vi "0926New Project.vi"() -> ()   [LabVIEW 2011] (continued)
      n72 = property on="S-para Pair Name" class="LstBox (严格)"("Value"=w56) -> ()  [unwired: 2 in, 2 out]
      n73 = property on="NEXT Pair Name" class="LstBox (严格)"("Value"=w56) -> ()  [unwired: 2 in, 2 out]
      n74 = property on="FEXT Pair Name" class="LstBox (严格)"("Value"=w56) -> ()  [unwired: 2 in, 2 out]
      n75 = property on="Single Test Items" class="LstBox (严格)"("Value"=w56) -> ()  [unwired: 2 in, 2 out]
      n76 = property on="FEXT Pair Name" class="LstBox (严格)"("Value"=w56) -> ()  [unwired: 2 in, 2 out]
      n77 = property on="Cable AWG:" class="Ring (严格)"("Value"=w56) -> ()  [unwired: 2 in, 2 out]
      n78 = property on="Customer" class="Ring (严格)"("Value"=w56) -> ()  [unwired: 2 in, 2 out]
      n79 = property on="TDR Test Items" class="LstBox (严格)"("Value"=w56) -> ()  [unwired: 2 in, 2 out]
      n80 = call <vilib>:"Application Directory.vi"() -> ("Application Directory"=w32:path)
      n81 = property on="Default" class="RadioBtnsControl (严格)"("Value"=w56) -> ()  [unwired: 2 in, 2 out]
      n82 = Build Path(base path=w32, name or relative path="template" ("名称或相对路径")) -> (appended path=w33:path)
      n83 = call "Get_initialize_Config.vi"() -> ("Local Database"=w24:bool)  [unwired: 11 in]
      n84 = local write "Report Templete Path:"(w33) -> ()
      n85 = local write "Local"(w24) -> ()
      n86 = property on="Excute" class="Bool"("DisabledEnum"=w29) -> ()  [unwired: 2 in, 2 out]
      n87 = property on="Query" class="Bool (严格)"("DisabledEnum"=w29) -> ()  [unwired: 2 in, 2 out]
      n88 = property on="Save" class="Bool (严格)"("DisabledEnum"=T4."Disabled and Grayed Out" ("禁用")) -> ()  [unwired: 2 in, 2 out]
      n89 = local write "Query"(FALSE ("Query")) -> ()
      n90 = local write "Update"(FALSE ("Query")) -> ()
      n91 = local write "Delete"(FALSE ("Query")) -> ()
      n92 = local write "Save"(FALSE ("Query")) -> ()
      n93 = property on="SNType" class="Str"("Visible"=w24) -> ()  [unwired: 2 in, 2 out]
      n94 = property on="CmdType" class="Ring (严格)"("Visible"=w24) -> ()  [unwired: 2 in, 2 out]
      n95 = property on="Update" class="Bool (严格)"("DisabledEnum"=T4."Disabled and Grayed Out" ("禁用")) -> ()  [unwired: 2 in, 2 out]
      n96 = property on="Delete" class="Bool (严格)"("DisabledEnum"=T4."Disabled and Grayed Out" ("禁用")) -> ()  [unwired: 2 in, 2 out]
      n97 = property on="Luxshare_P/N:" class="Str"("DisabledEnum"=T4."Disabled and Grayed Out" ("禁用")) -> ()  [unwired: 2 in, 2 out]
      "midVar_bool_timStop" <- FALSE ("midVar_bool_timStop")
    }
    frame #2 {
      n98 = while {
        stop <- w104 stop-if-true
        n99 = local read "midVar_timeStart"() -> (w103:timestamp)
        n100 = local read "midVar_bool_timStop"() -> (w104:bool)
        n101 = Get Date/Time In Seconds() -> (seconds since 1Jan1904=w105:timestamp)
        n102 = Subtract(x=w105, y=w103) -> (x-y=→"访问DB(s)":dbl)
      }
      n103 = call <vilib>:"System Exec.vi"("run minimized? (F)"=TRUE, "wait until completion? (T)"=TRUE, "command line"="ping DG-MESDB.luxshare.com.cn") -> ("standard output"=w96:string)  [unwired: 5 in, 3 out]
      n104 = Search and Replace String(replace all?=TRUE ("替换全部？(F)"), case sensitive?=TRUE ("忽略大小写？(F)"), input string=w96, search string="TTL" ("搜索字符串")) -> (number of replacements=w98:i32)  [unwired: 4 in, 3 out]
      n105 = Greater Than 0?(x=w98) -> (x > 0?=w93:bool)
      n106 = case shown="真" w93 {
        frame False {
          w109 = T4."Enabled" ("禁用")
          # "连不上数据库，local禁用，默认勾选"
          n107 = property on="Query" class="Bool (严格)"("DisabledEnum"=w109) -> ()  [unwired: 2 in, 2 out]
          n108 = property on="Save" class="Bool (严格)"("DisabledEnum"=w109) -> ()  [unwired: 2 in, 2 out]
          n109 = local write "midVar_bool_timStop"(TRUE ("midVar_bool_timStop")) -> ()
          n110 = One Button Dialog(message="fail to connect DB!\nyou can use local DB only!") -> ()  [unwired: 1 in, 1 out]
          n111 = property on="Excute" class="Bool"("DisabledEnum"=w109) -> ()  [unwired: 2 in, 2 out]
          n112 = property on="Local" class="Bool (严格)"("DisabledEnum"=T4."Disabled and Grayed Out" ("禁用")) -> ()  [unwired: 2 in, 2 out]
          n113 = local write "Local"(TRUE ("Local")) -> ()
          n114 = property on="FixtureNo" class="CmbBox"("Strings And Values[]"=T5 [{"String"="No Data", "Value"="No Data"}] ("字符串与值[]")) -> ()  [unwired: 2 in, 2 out]
          n115 = property on="FixtureNo" class="CmbBox"("DisabledEnum"=T4."Disabled and Grayed Out" ("禁用")) -> ()  [unwired: 2 in, 2 out]
        }
        frame True {
          n116 = stacked-sequence {
            frame #0 {
              w114 = T4."Enabled" ("禁用")
              w113 = T4."Enabled" ("禁用")
              n117 = property on="Local" class="Bool (严格)"("DisabledEnum"=w113) -> ()  [unwired: 2 in, 2 out]
              n118 = property on="Query" class="Bool (严格)"("DisabledEnum"=w113) -> ()  [unwired: 2 in, 2 out]
              n119 = property on="Save" class="Bool (严格)"("DisabledEnum"=w114) -> ()  [unwired: 2 in, 2 out]
              n120 = property on="Excute" class="Bool"("DisabledEnum"=w114) -> ()  [unwired: 2 in, 2 out]
            }
            frame #1 {
              n121 = call "sql-readinfo_vfixture.vi"("操作模式"=T6."查询数据", "查询项目"="FixtureNo", "限定条件"="") -> ("ConvertToArray"=w119:string[][], "ResultString"=w118:string)  [unwired: 14 in, 9 out]
              n122 = call <vilib>:"Trim Whitespace.vi"("string"=w118) -> ("trimmed string"=w117:string)  [unwired: 1 in]
              n123 = Empty String/Path?(string/path=w117) -> (empty?=w116:bool)
              n124 = case shown="假" w116 {
                tunnel: w119 -> [w126 _]
                frame False {
                  n125 = Index Array(array=w126, index (col)=0 ("索引 (行)")) -> (element=w125:string[])  [unwired: 1 in]
                  n126 = for {
                    tunnel: w125 -> [w128] mode=indexing
                    tunnel: [w127] -> w124 mode=indexing
                    n127 = Bundle("字符串"=w128, "字符串"=w128) -> (w127:cluster{"字符串":string, "字符串":string})  [unwired: 1 in]
                  }
                  n128 = property on="FixtureNo" class="CmbBox"("Strings And Values[]"=w124) -> ()  [unwired: 2 in, 2 out]
                  n129 = property on="FixtureNo" class="CmbBox"("DisabledEnum"=T4."Enabled" ("禁用")) -> ()  [unwired: 2 in, 2 out]
                }
                frame True {
                  n130 = property on="FixtureNo" class="CmbBox"("Strings And Values[]"=T5 [{"String"="No Data", "Value"="No Data"}] ("字符串与值[]")) -> ()  [unwired: 2 in, 2 out]
                  n131 = property on="FixtureNo" class="CmbBox"("DisabledEnum"=T4."Disabled and Grayed Out" ("禁用")) -> ()  [unwired: 2 in, 2 out]
                }
              }
            }
            frame #2 {
              n132 = local write "midVar_bool_timStop"(TRUE ("midVar_bool_timStop")) -> ()
            }
          }
        }
      }
    }
    frame #3 {
      n133 = control-ref of="Label Num"() -> (w132:refnum<vi>)
      n134 = control-ref of="FixtureNo"() -> (w155:refnum<vi>)
      n135 = control-ref of="Label Num"() -> (w154:refnum<vi>)
      n136 = control-ref of="Label Content"() -> (w153:refnum<vi>)
      n137 = control-ref of="SNType"() -> (w152:refnum<vi>)
      n138 = control-ref of="Customer_P/N:"() -> (w162:refnum<vi>)
      n139 = control-ref of="Length(mm):"() -> (w161:refnum<vi>)
      n140 = control-ref of="Sample Description:"() -> (w160:refnum<vi>)
      n141 = control-ref of="Remark:"() -> (w159:refnum<vi>)
      n142 = control-ref of="Switch Matrix"() -> (w158:refnum<vi>)
      n143 = control-ref of="VNA Cal File Path:"() -> (w156:refnum<vi>)
      n144 = control-ref of="EEPROM Write/Read ?"() -> (w151:refnum<vi>)
      n145 = control-ref of="Label Print?"() -> (w150:refnum<vi>)
      n146 = Build Array(w151, w150) -> (→"bool":refnum<vi>[])
      n147 = Build Array(w156, w162, w161, w160, w159, w158, w155, w154, w153, w132, w152) -> (→"string":refnum<vi>[])
      n148 = control-ref of="Spec Associate"() -> (w148:refnum<vi>)
      n149 = control-ref of="Postion for Raw data"() -> (w147:refnum<vi>)
      n150 = control-ref of="Impedance Spec:"() -> (w133:refnum<vi>)
      n151 = control-ref of="Start TimeNs"() -> (w146:refnum<vi>)
      n152 = control-ref of="StopTimeNs"() -> (w145:refnum<vi>)
      n153 = control-ref of="Filter Risetime(ps)"() -> (w144:refnum<vi>)
      n154 = control-ref of="Compensation(ohm)"() -> (w143:refnum<vi>)
      n155 = Build Array(w133, w148, w147) -> (→"chart":refnum<vi>[])
      n156 = Build Array(w146, w145, w144, w143) -> (→"number":refnum<vi>[])
      n157 = control-ref of="Diff Test Items"() -> (w142:refnum<vi>)
      n158 = control-ref of="Single Test Items"() -> (w141:refnum<vi>)
      n159 = control-ref of="TDR Test Items"() -> (w140:refnum<vi>)
      n160 = control-ref of="S-para Pair Name"() -> (w139:refnum<vi>)
      n161 = control-ref of="NEXT Pair Name"() -> (w138:refnum<vi>)
      n162 = control-ref of="FEXT Pair Name"() -> (w137:refnum<vi>)
      n163 = Build Array(w142, w141, w140, w139, w138, w137) -> (→"list":refnum<vi>[])
      n164 = property on="访问DB(s)" class="DigNum (严格)"("Visible"=FALSE ("可见")) -> ()  [unwired: 2 in, 2 out]
    }
    frame #4 {
      n165 = while {
        stop <- w165 stop-if-true
        n166 = event shown="[17] \"Excute\": 值改变" {
          selector: _ -> [_ _ _ _ _ _ _ _ _ _ _ _ _ _ _ _ _ _ _ _ _ _ _]
          dyn-events: _ -> [_ _ _ _ _ _ _ _ _ _ _ _ _ _ _ _ _ _ _ _ _ _ _]
          timeout: 500 -> [_ _ _ _ _ _ _ _ _ _ _ _ _ _ _ _ _ _ _ _ _ _ _]
          tunnel: [_ _ _ _ _ _ _ _ _ _ _ _ _ _ _ _ _ _ _ TRUE _ _ _] -> w165
          event Timeout {
            n167 = event-data() -> ()  [unwired: 1 in, 2 out]
          }
          event "Length(mm):", "VNA Cal File Path:", "Switch Matrix", "Luxshare_P/N:": Value Change {
            n168 = event-data() -> ()  [unwired: 1 in, 5 out]
          }
          event "Local": Value Change {
            n169 = event-data() -> ()  [unwired: 1 in, 5 out]
            n170 = local read "Local"() -> (w166:bool)
            n171 = Not(x=w166) -> (.not. x?=w167:bool)
            n172 = property on="SNType" class="Str"("Visible"=w166) -> ()  [unwired: 2 in, 2 out]
            n173 = property on="CmdType" class="Ring (严格)"("Visible"=w166) -> ()  [unwired: 2 in, 2 out]
            n174 = property on="System_Mode" class="Ring (严格)"("Visible"=w167) -> ()  [unwired: 2 in, 2 out]
          }
          event "Quick": Value Change {
            n175 = event-data() -> ("NewVal"=w170:bool)  [unwired: 1 in, 4 out]
            n176 = Equal?(x=w170, y=TRUE) -> (x = y?=w168:bool)
            n177 = case shown="真" w168 {
              frame False {
                n178 = property on="Postion for Raw data" class="Tbl (严格)"("Value"=string[][] [] ("Postion for Raw data")) -> ()  [unwired: 2 in, 2 out]
              }
              frame True {
                w173 = T3 {"Row"=0, "Column"=0} ("编辑位置")
                w174 = u32 4 ("列数")
                n179 = property on="Single Test Items" class="LstBox (严格)"() -> ("Item Names"=w191:string[], "Item Symbols"=w190:i32[])  [unwired: 2 in, 2 out]
                n180 = property on="TDR Test Items" class="LstBox (严格)"() -> ("Item Names"=w189:string[], "Item Symbols"=w188:i32[])  [unwired: 2 in, 2 out]
                n181 = property on="Diff Test Items" class="LstBox (严格)"() -> ("Item Names"=w193:string[], "Item Symbols"=w192:i32[])  [unwired: 2 in, 2 out]
                n182 = call "_wmg_SelectItems2.vi"("Item Syms"=w188, "Item name"=w189) -> ("Selected tem"=w187:string[])  [unwired: 7 in, 2 out]
                n183 = call "_wmg_SelectItems2.vi"("Item Syms"=w192, "Item name"=w193) -> ("Selected tem"=w186:string[])  [unwired: 7 in, 2 out]
                n184 = call "_wmg_SelectItems2.vi"("Item Syms"=w190, "Item name"=w191) -> ("Selected tem"=w185:string[])  [unwired: 7 in, 2 out]
                n185 = Insert Into Array(array=w187, new element #1=w186, new element #2=w185) -> (w182:string[])  [unwired: 1 in]
                n186 = Array Size(array=w182) -> (size(s)=w179:i32)
                n187 = for {
                  N: w179 -> [_]
                  tunnel: [w194] -> w183 mode=indexing
                  i -> [w195]
                  n188 = Increment(x=w195) -> (x+1=w194:i32)
                }
                n189 = Initialize Array("2", w179) -> (w177:string[])
                n190 = Initialize Array("0", w179) -> (w176:string[])
                n191 = Number To Decimal String(number=w183) -> (decimal integer string=w181:string[])  [unwired: 1 in]
                n192 = Build Array(w182, w181, w177, w176) -> (w175:string[][])
                n193 = Transpose 2D Array(2D array=w175) -> (transposed array=w184:string[][])
                n194 = property on="Postion for Raw data" class="Tbl (严格)"("Value"=w184, "EditPos"=T3 {"Row"=0, "Column"=0} ("编辑位置")) -> ()  [unwired: 2 in, 2 out]
                n195 = property on="Postion for Raw data" class="Tbl (严格)"("Number of Columns"=w174, "EditPos"=w173) -> ()  [unwired: 2 in, 2 out]
                n196 = property on="Postion for \"PN&Tester&Date\" etc Fields" class="Tbl (严格)"("Number of Columns"=w174, "EditPos"=w173) -> ()  [unwired: 2 in, 2 out]
              }
            }
          }
          event "Diff Test Items": Double Click {
            n197 = event-data() -> ("Row"=w196:i32)  [unwired: 1 in, 7 out]
            n198 = stacked-sequence {
              tunnel: w196 -> [w203 _ _]
              frame #0 {
                w200 = 38 ("y")
                n199 = property on="Diff Test Items" class="LstBox (严格)"() -> ("Item Symbols"=w204:i32[])  [unwired: 2 in, 2 out]
                n200 = Index Array(array=w204, index=w203) -> (element=w202:i32)
                n201 = Equal?(x=w202, y=w200) -> (x = y?=w201:bool)
                n202 = Select(t=37, s=w201, f=w200) -> (s? t:f=w198:i32)
                n203 = Replace Array Subset(array=w204, new element=w198, index=w203) -> (w197:i32[])
                n204 = property on="Diff Test Items" class="LstBox (严格)"("Item Symbols"=w197) -> ()  [unwired: 2 in, 2 out]
              }
              frame #1 {
                n205 = property on="Postion for Raw data" class="Tbl (严格)"("Value"=string[][] [] ("Postion for Raw data"), "EditPos"=T3 {"Row"=0, "Column"=0} ("编辑位置")) -> ()  [unwired: 2 in, 2 out]
              }
              frame #2 {
                w208 = T3 {"Row"=0, "Column"=0} ("编辑位置")
                w209 = u32 4 ("列数")
                n206 = property on="Single Test Items" class="LstBox (严格)"() -> ("Item Names"=w226:string[], "Item Symbols"=w225:i32[])  [unwired: 2 in, 2 out]
                n207 = property on="TDR Test Items" class="LstBox (严格)"() -> ("Item Names"=w224:string[], "Item Symbols"=w223:i32[])  [unwired: 2 in, 2 out]
                n208 = property on="Diff Test Items" class="LstBox (严格)"() -> ("Item Names"=w228:string[], "Item Symbols"=w227:i32[])  [unwired: 2 in, 2 out]
                n209 = property on="Postion for Raw data" class="Tbl (严格)"("Number of Columns"=w209, "EditPos"=w208) -> ()  [unwired: 2 in, 2 out]
                n210 = property on="Postion for \"PN&Tester&Date\" etc Fields" class="Tbl (严格)"("Number of Columns"=w209, "EditPos"=w208) -> ()  [unwired: 2 in, 2 out]
                n211 = call "_wmg_SelectItems2.vi"("Item Syms"=w223, "Item name"=w224) -> ("Selected tem"=w222:string[])  [unwired: 7 in, 2 out]
                n212 = call "_wmg_SelectItems2.vi"("Item Syms"=w227, "Item name"=w228) -> ("Selected tem"=w221:string[])  [unwired: 7 in, 2 out]
                n213 = call "_wmg_SelectItems2.vi"("Item Syms"=w225, "Item name"=w226) -> ("Selected tem"=w220:string[])  [unwired: 7 in, 2 out]
                n214 = Insert Into Array(array=w222, new element #1=w221, new element #2=w220) -> (w217:string[])  [unwired: 1 in]
                n215 = Array Size(array=w217) -> (size(s)=w214:i32)
                n216 = for {
                  N: w214 -> [_]
                  tunnel: [w229] -> w218 mode=indexing
                  i -> [w230]
                  n217 = Increment(x=w230) -> (x+1=w229:i32)
                }
                n218 = Initialize Array("2", w214) -> (w212:string[])
                n219 = Initialize Array("0", w214) -> (w211:string[])
                n220 = Number To Decimal String(number=w218) -> (decimal integer string=w216:string[])  [unwired: 1 in]
                n221 = Build Array(w217, w216, w212, w211) -> (w210:string[][])
                n222 = Transpose 2D Array(2D array=w210) -> (transposed array=w219:string[][])
                n223 = property on="Postion for Raw data" class="Tbl (严格)"("Value"=w219, "EditPos"=T3 {"Row"=0, "Column"=0} ("编辑位置")) -> ()  [unwired: 2 in, 2 out]
              }
            }
          }
          event "TDR Test Items": Double Click {
            n224 = event-data() -> ("Row"=w231:i32)  [unwired: 1 in, 7 out]
            n225 = stacked-sequence {
              tunnel: w231 -> [w239 _ _]
              frame #0 {
                w236 = 38 ("y")
                n226 = property on="TDR Test Items" class="LstBox (严格)"() -> ("Item Symbols"=w233:i32[])  [unwired: 2 in, 2 out]
                n227 = Index Array(array=w233, index=w239) -> (element=w238:i32)
                n228 = Equal?(x=w238, y=w236) -> (x = y?=w237:bool)
                n229 = Select(t=37, s=w237, f=w236) -> (s? t:f=w234:i32)
                n230 = Replace Array Subset(array=w233, new element=w234, index=w239) -> (w232:i32[])
                n231 = property on="TDR Test Items" class="LstBox (严格)"("Item Symbols"=w232) -> ()  [unwired: 2 in, 2 out]
              }
              frame #1 {
                n232 = property on="Postion for Raw data" class="Tbl (严格)"("Value"=string[][] [] ("Postion for Raw data"), "EditPos"=T3 {"Row"=0, "Column"=0} ("编辑位置")) -> ()  [unwired: 2 in, 2 out]
              }
              frame #2 {
                w243 = T3 {"Row"=0, "Column"=0} ("编辑位置")
                w244 = u32 4 ("列数")
                n233 = property on="Single Test Items" class="LstBox (严格)"() -> ("Item Names"=w261:string[], "Item Symbols"=w260:i32[])  [unwired: 2 in, 2 out]
                n234 = property on="TDR Test Items" class="LstBox (严格)"() -> ("Item Names"=w259:string[], "Item Symbols"=w258:i32[])  [unwired: 2 in, 2 out]
                n235 = property on="Diff Test Items" class="LstBox (严格)"() -> ("Item Names"=w263:string[], "Item Symbols"=w262:i32[])  [unwired: 2 in, 2 out]
                n236 = property on="Postion for Raw data" class="Tbl (严格)"("Number of Columns"=w244, "EditPos"=w243) -> ()  [unwired: 2 in, 2 out]
                n237 = property on="Postion for \"PN&Tester&Date\" etc Fields" class="Tbl (严格)"("Number of Columns"=w244, "EditPos"=w243) -> ()  [unwired: 2 in, 2 out]
                n238 = call "_wmg_SelectItems2.vi"("Item Syms"=w258, "Item name"=w259) -> ("Selected tem"=w257:string[])  [unwired: 7 in, 2 out]
                n239 = call "_wmg_SelectItems2.vi"("Item Syms"=w262, "Item name"=w263) -> ("Selected tem"=w256:string[])  [unwired: 7 in, 2 out]
                n240 = call "_wmg_SelectItems2.vi"("Item Syms"=w260, "Item name"=w261) -> ("Selected tem"=w255:string[])  [unwired: 7 in, 2 out]
                n241 = Insert Into Array(array=w257, new element #1=w256, new element #2=w255) -> (w252:string[])  [unwired: 1 in]
                n242 = Array Size(array=w252) -> (size(s)=w249:i32)
                n243 = for {
                  N: w249 -> [_]
                  tunnel: [w264] -> w253 mode=indexing
                  i -> [w265]
                  n244 = Increment(x=w265) -> (x+1=w264:i32)
                }
                n245 = Initialize Array("2", w249) -> (w247:string[])
                n246 = Initialize Array("0", w249) -> (w246:string[])
                n247 = Number To Decimal String(number=w253) -> (decimal integer string=w251:string[])  [unwired: 1 in]
                n248 = Build Array(w252, w251, w247, w246) -> (w245:string[][])
                n249 = Transpose 2D Array(2D array=w245) -> (transposed array=w254:string[][])
                n250 = property on="Postion for Raw data" class="Tbl (严格)"("Value"=w254, "EditPos"=T3 {"Row"=0, "Column"=0} ("编辑位置")) -> ()  [unwired: 2 in, 2 out]
              }
            }
          }
          event "S-para Pair Name": Double Click {
            w270 = 38 ("y")
            n251 = event-data() -> ("Row"=w266:i32)  [unwired: 1 in, 7 out]
            n252 = property on="S-para Pair Name" class="LstBox (严格)"() -> ("Item Symbols"=w273:i32[])  [unwired: 2 in, 2 out]
            n253 = Index Array(array=w273, index=w266) -> (element=w272:i32)
            n254 = Equal?(x=w272, y=w270) -> (x = y?=w271:bool)
            n255 = Select(t=37, s=w271, f=w270) -> (s? t:f=w268:i32)
            n256 = Replace Array Subset(array=w273, new element=w268, index=w266) -> (w267:i32[])
            n257 = property on="S-para Pair Name" class="LstBox (严格)"("Item Symbols"=w267) -> ()  [unwired: 2 in, 2 out]
          }
          event "NEXT Pair Name": Double Click {
            w278 = 38 ("y")
            n258 = event-data() -> ("Row"=w274:i32)  [unwired: 1 in, 7 out]
            n259 = property on="NEXT Pair Name" class="LstBox (严格)"() -> ("Item Symbols"=w281:i32[])  [unwired: 2 in, 2 out]
            n260 = Index Array(array=w281, index=w274) -> (element=w280:i32)
            n261 = Equal?(x=w280, y=w278) -> (x = y?=w279:bool)
            n262 = Select(t=37, s=w279, f=w278) -> (s? t:f=w276:i32)
            n263 = Replace Array Subset(array=w281, new element=w276, index=w274) -> (w275:i32[])
            n264 = property on="NEXT Pair Name" class="LstBox (严格)"("Item Symbols"=w275) -> ()  [unwired: 2 in, 2 out]
          }
          event "FEXT Pair Name": Double Click {
            w282 = 38 ("y")
            n265 = event-data() -> ("Row"=w283:i32)  [unwired: 1 in, 7 out]
            n266 = property on="FEXT Pair Name" class="LstBox (严格)"() -> ("Item Symbols"=w289:i32[])  [unwired: 2 in, 2 out]
            n267 = Index Array(array=w289, index=w283) -> (element=w288:i32)
            n268 = Equal?(x=w288, y=w282) -> (x = y?=w287:bool)
            n269 = Select(t=37, s=w287, f=w282) -> (s? t:f=w285:i32)
            n270 = Replace Array Subset(array=w289, new element=w285, index=w283) -> (w284:i32[])
            n271 = property on="FEXT Pair Name" class="LstBox (严格)"("Item Symbols"=w284) -> ()  [unwired: 2 in, 2 out]
          }
          event "Single Test Items": Double Click {
            n272 = event-data() -> ("Row"=w290:i32)  [unwired: 1 in, 7 out]
            n273 = stacked-sequence {
              tunnel: w290 -> [w292 _ _]
              frame #0 {
                w291 = 38 ("y")
                n274 = property on="Single Test Items" class="LstBox (严格)"() -> ("Item Symbols"=w298:i32[])  [unwired: 2 in, 2 out]
                n275 = Index Array(array=w298, index=w292) -> (element=w297:i32)
                n276 = Equal?(x=w297, y=w291) -> (x = y?=w296:bool)
                n277 = Select(t=37, s=w296, f=w291) -> (s? t:f=w294:i32)
                n278 = Replace Array Subset(array=w298, new element=w294, index=w292) -> (w293:i32[])
                n279 = property on="Single Test Items" class="LstBox (严格)"("Item Symbols"=w293) -> ()  [unwired: 2 in, 2 out]
              }
              frame #1 {
                n280 = property on="Postion for Raw data" class="Tbl (严格)"("Value"=string[][] [] ("Postion for Raw data"), "EditPos"=T3 {"Row"=0, "Column"=0} ("编辑位置")) -> ()  [unwired: 2 in, 2 out]
              }
              frame #2 {
                w302 = T3 {"Row"=0, "Column"=0} ("编辑位置")
                w303 = u32 4 ("列数")
                n281 = property on="Single Test Items" class="LstBox (严格)"() -> ("Item Names"=w320:string[], "Item Symbols"=w319:i32[])  [unwired: 2 in, 2 out]
                n282 = property on="TDR Test Items" class="LstBox (严格)"() -> ("Item Names"=w318:string[], "Item Symbols"=w317:i32[])  [unwired: 2 in, 2 out]
                n283 = property on="Diff Test Items" class="LstBox (严格)"() -> ("Item Names"=w322:string[], "Item Symbols"=w321:i32[])  [unwired: 2 in, 2 out]
                n284 = property on="Postion for Raw data" class="Tbl (严格)"("Number of Columns"=w303, "EditPos"=w302) -> ()  [unwired: 2 in, 2 out]
                n285 = property on="Postion for \"PN&Tester&Date\" etc Fields" class="Tbl (严格)"("Number of Columns"=w303, "EditPos"=w302) -> ()  [unwired: 2 in, 2 out]
                n286 = call "_wmg_SelectItems2.vi"("Item Syms"=w317, "Item name"=w318) -> ("Selected tem"=w316:string[])  [unwired: 7 in, 2 out]
                n287 = call "_wmg_SelectItems2.vi"("Item Syms"=w321, "Item name"=w322) -> ("Selected tem"=w315:string[])  [unwired: 7 in, 2 out]
                n288 = call "_wmg_SelectItems2.vi"("Item Syms"=w319, "Item name"=w320) -> ("Selected tem"=w314:string[])  [unwired: 7 in, 2 out]
                n289 = Insert Into Array(array=w316, new element #1=w315, new element #2=w314) -> (w311:string[])  [unwired: 1 in]
                n290 = Array Size(array=w311) -> (size(s)=w308:i32)
                n291 = for {
                  N: w308 -> [_]
                  tunnel: [w323] -> w312 mode=indexing
                  i -> [w324]
                  n292 = Increment(x=w324) -> (x+1=w323:i32)
                }
                n293 = Initialize Array("2", w308) -> (w306:string[])
                n294 = Initialize Array("0", w308) -> (w305:string[])
                n295 = Number To Decimal String(number=w312) -> (decimal integer string=w310:string[])  [unwired: 1 in]
                n296 = Build Array(w311, w310, w306, w305) -> (w304:string[][])
                n297 = Transpose 2D Array(2D array=w304) -> (transposed array=w313:string[][])
                n298 = property on="Postion for Raw data" class="Tbl (严格)"("Value"=w313, "EditPos"=T3 {"Row"=0, "Column"=0} ("编辑位置")) -> ()  [unwired: 2 in, 2 out]
              }
            }
          }
          event "Import Spec": Value Change {
            n299 = event-data() -> ()  [unwired: 1 in, 5 out]
            n300 = case shown="真" "Import Spec" {
              frame False {
              }
              frame True {
                n301 = call <vilib>:"Application Directory.vi"() -> ("Application Directory"=w328:path)
                n302 = Build Path(base path=w328, name or relative path="Spec" ("名称或相对路径")) -> (appended path=w326:path)
                n303 = call "文件对话框"("start path"=w326) -> ("selected path"=w330:path, "error out"=w329:errorcluster)  [unwired: 11 in, 2 out]
                n304 = case shown="无错误" w329 {
                  tunnel: w330 -> [w331 _]
                  frame No Error {
                    n305 = stacked-sequence {
                      tunnel: w331 -> [_ w359]
                      frame #0 {
                        n306 = property on="Diff Test Items" class="LstBox (严格)"() -> ("Item Symbols"=w338:i32[], "Item Names"=w336:string[])  [unwired: 2 in, 2 out]
                        n307 = for {
                          tunnel: w338 -> [w349] mode=indexing
                          shift-right: [w344] -> w334
                          shift-left: string[] [] -> [w345]
                          tunnel: w336 -> [w346] mode=indexing
                          shift-right: [w343] -> w333
                          shift-left: string[] [] -> [w342]
                          n308 = Array Size(array=w342) -> (size(s)=w341:i32)
                          n309 = Equal?(x=w349, y=38) -> (x = y?=w347:bool)
                          n310 = Increment(x=w341) -> (x+1=w340:i32)
                          n311 = Number To Decimal String(number=w340) -> (decimal integer string=w339:string)  [unwired: 1 in]
                          n312 = case shown="真" w347 {
                            tunnel: w346 -> [_ w357]
                            tunnel: w345 -> [w351 w356]
                            tunnel: [w351 w355] -> w344
                            tunnel: w342 -> [w350 w354]
                            tunnel: [w350 w353] -> w343
                            tunnel: w339 -> [_ w352]
                            frame False {
                            }
                            frame True {
                              n313 = Insert Into Array(array=w354, new element=w352) -> (w353:string[])  [unwired: 1 in]
                              n314 = Insert Into Array(array=w356, new element=w357) -> (w355:string[])  [unwired: 1 in]
                            }
                          }
                        }
                        n315 = Build Array(w334, w333) -> (w332:string[][])
                        n316 = local write "Spec Associate"(w332) -> ()
                      }
                      frame #1 {
                        n317 = Path To String(path=w359) -> (string=w358:string)
                        n318 = call "Import Spec From Excel.vi"("Spec Path"=w359) -> ("Spec _Data"=w365:dbl[][])  [unwired: 26 in]
                        n319 = Array Subset(array=w365, length (row)="Spec Points") -> (w360:dbl[][])  [unwired: 3 in]
                        n320 = local write "Spec File Path"(w358) -> ()
                        n321 = local write "Spec _Data"(w360) -> ()
                        n322 = Array To Spreadsheet String(delimiter (Tab)="#" ("分隔符(Tab)"), array=w360, 3:"%s" ("格式字符串")) -> (spreadsheet string=→"Spec String":string)
                      }
                    }
                  }
                  frame Error {
                  }
                }
              }
            }
          }
          event "From File": Value Change {
            n323 = event-data() -> ()  [unwired: 1 in, 5 out]
            n324 = case shown="假" "From File" {
              tunnel: [2 0] -> w366
              frame False {
              }
              frame True {
              }
            }
            n325 = property on="Import_FixS4P" class="Bool"("DisabledEnum"=w366) -> ()  [unwired: 2 in, 2 out]
          }
          event "FixtureType": Value Change {
            n326 = event-data() -> ()  [unwired: 1 in, 5 out]
            n327 = local read "FixtureNo"() -> (w371:string)
            n328 = Search and Replace String(input string=" where FixtureNo='@' " ("限定条件"), search string="@" ("搜索字符串"), replace string=w371) -> (result string=w370:string)  [unwired: 5 in, 3 out]
            n329 = call "sql-readinfo_vfixture.vi"("操作模式"=T6."查询数据", "查询项目"=" S4P10G,S4P20G,S4P27G,S4P40G ", "限定条件"=w370) -> ("ConvertToArray"=w378:string[][], "ResultString"=w377:string)  [unwired: 14 in, 9 out]
            n330 = call <vilib>:"Trim Whitespace.vi"("string"=w377) -> ("trimmed string"=w376:string)  [unwired: 1 in]
            n331 = Empty String/Path?(string/path=w376) -> (empty?=w375:bool)
            n332 = case shown="假" w375 {
              tunnel: w378 -> [w384 _]
              frame False {
                n333 = Index Array(array=w384, index (col)=0 ("索引 (行)")) -> (element=w383:string[])  [unwired: 1 in]
                n334 = for {
                  tunnel: w383 -> [w386] mode=indexing
                  tunnel: [w385] -> w382 mode=indexing
                  n335 = Bundle("字符串"=w386, "字符串"=w386) -> (w385:cluster{"字符串":string, "字符串":string})  [unwired: 1 in]
                }
                n336 = property on="FixtureNo" class="CmbBox"("Strings And Values[]"=w382) -> ()  [unwired: 2 in, 2 out]
                n337 = property on="FixtureNo" class="CmbBox"("DisabledEnum"=T4."Enabled" ("禁用")) -> ()  [unwired: 2 in, 2 out]
              }
              frame True {
                n338 = property on="FixtureNo" class="CmbBox"("Strings And Values[]"=T5 [{"String"="No Data", "Value"="No Data"}] ("字符串与值[]")) -> ()  [unwired: 2 in, 2 out]
                n339 = property on="FixtureNo" class="CmbBox"("DisabledEnum"=T4."Disabled and Grayed Out" ("禁用")) -> ()  [unwired: 2 in, 2 out]
              }
            }
          }
          event "Import_FixS4P": Value Change {
            n340 = event-data() -> ()  [unwired: 1 in, 5 out]
            n341 = case shown="真" "Import_FixS4P" {
              frame False {
              }
              frame True {
                n342 = call "文件对话框3"("pattern (all files)"="*.s4p" ("DNL"), "pattern label"="SnP文件") -> ("selected path"=w391:path, "exists"=w392:bool)  [unwired: 10 in, 2 out]
                n343 = case shown="真" w392 {
                  tunnel: w391 -> [_ w396]
                  tunnel: "Port Type" -> [_ w395]
                  frame False {
                  }
                  frame True {
                    n344 = stacked-sequence {
                      tunnel: w396 -> [_ w407 w420 _]
                      tunnel: w395 -> [_ w402 w418 _]
                      frame #0 {
                        n345 = property on="Import_FixS4P" class="Bool"("DisabledEnum"=2) -> ()  [unwired: 2 in, 2 out]
                      }
                      frame #1 {
                        n346 = call "S4P to Sparameter.vi"("S4P File Path"=w407, "Port Type"=w402) -> ("Frequency(Hz)"=w404:dbl[], "Diff S-parameters Data"=w406:dbl[][])  [unwired: 14 in, 2 out]
                        n347 = Index Array(array=w406, index (row)=0 ("索引 (行)")) -> (element=w400:dbl[])  [unwired: 1 in]
                        "2X Thru  IL Data" <- w400
                        n348 = Bundle("Frequency(Hz)"=w404, "Diff S-parameters Data"=w400) -> (w403:T2)  [unwired: 1 in]
                        n349 = local write "Insertion Loss"(w403) -> ()
                        n350 = Array To Spreadsheet String(array=w400, 3:"%s" ("格式字符串")) -> (spreadsheet string=w399:string)  [unwired: 1 in]
                        n351 = call <vilib>:"Trim Whitespace.vi"("string"=w399) -> ("trimmed string"=→"2X Thru String":string)  [unwired: 1 in]
                      }
                      frame #2 {
                        w423 = i16 2 items=["StepReal", "ImpulseReal", "StepVolts", "ImpulseVolts", "StepLog", "ImpulseLog", "StepImpedance"] ("dataFormat")
                        n352 = Path To String(path=w420) -> (string=w419:string)
                        n353 = call "Export_TimeDomain_Data.vi"("szFileName"=w419, "dataFormat"=w423, "stopTimeNs"=1.6, "ParamList"="TDD21", "Port Type"=w418, "startTimeNs"=0.0) -> ("Data Out"=w417:dbl[][], "Time Array"=w410:dbl[])  [unwired: 20 in]
                        n354 = Index Array(array=w417, index (row)=0 ("索引 (行)")) -> (element=w413:dbl[])  [unwired: 1 in]
                        "2X Delay Data" <- w413
                        n355 = Threshold 1D Array(2:0.2 ("过阈值的y"), 3:w413) -> (0:w411:dbl)  [unwired: 1 in]
                        n356 = To Long Integer(number=w411) -> (32bit integer=w409:i32)
                        n357 = Bundle("Time Array"=w410, "Data Out"=w413) -> (w415:cluster{"Time Array":dbl[], "Data Out":dbl[]})  [unwired: 1 in]
                        n358 = Index Array(array=w410, index=w409) -> (element=→"Delay(ns)":dbl)
                        n359 = local write "Delay"(w415) -> ()
                      }
                      frame #3 {
                        n360 = property on="Import_FixS4P" class="Bool"("DisabledEnum"=0) -> ()  [unwired: 2 in, 2 out]
                      }
                    }
                  }
                }
              }
            }
          }
          event "Import Matrix?": Value Change {
            n361 = event-data() -> ()  [unwired: 1 in, 5 out]
            n362 = case shown="真" "Import Matrix?" {
              frame False {
              }
              frame True {
                n363 = call <vilib>:"Application Directory.vi"() -> ("Application Directory"=w428:path)
                n364 = Build Path(base path=w428, name or relative path="Switch Matrix" ("名称或相对路径")) -> (appended path=w426:path)
                n365 = call "文件对话框2"("start path"=w426) -> ("selected path"=w429:path, "error out"=w430:errorcluster)  [unwired: 11 in, 2 out]
                n366 = case shown="无错误" w430 {
                  tunnel: w429 -> [w432 _]
                  frame No Error {
                    n367 = Path To String(path=w432) -> (string=w431:string)
                    n368 = call-poly <vilib>:"Read From Spreadsheet File.vi"("format (%s)"="%s" ("format (%.3f)"), "file path (dialog if empty)"=w432) -> ("all rows"=w436:string[][])  [unwired: 5 in, 4 out]
                    n369 = Array To Spreadsheet String(delimiter (Tab)="#" ("分隔符(Tab)"), array=w436, 3:"%s" ("格式字符串")) -> (spreadsheet string=w433:string)
                    n370 = local write "Switch File Path"(w431) -> ()
                    n371 = local write "Switch Matrix"(w433) -> ()
                  }
                  frame Error {
                  }
                }
              }
            }
          }
          event "Impedance Spec:": Value Change {
            n372 = event-data() -> ()  [unwired: 1 in, 5 out]
            n373 = local read "Impedance Spec:"() -> (w438:string[][])
            n374 = call "impedance spec.vi"("Impedance Spec:"=w438) -> ("Impedance spec string"=→"Impedance spec string":string)  [unwired: 10 in]
          }
          event "Query", "Update", "Delete", "Save": Value Change {
            n375 = event-data() -> ("CtlRef"=w441:refnum<vi>)  [unwired: 1 in, 4 out]
            n376 = property class="Bool (严格)"(reference=w441) -> ("Label.Text"=w440:string)  [unwired: 1 in, 2 out]
            n377 = case shown="\"Save\"" w440 {
              frame "", Default {
                n378 = local write "Query"(FALSE ("Query")) -> ()
                n379 = local write "Update"(FALSE ("Update")) -> ()
                n380 = local write "Delete"(FALSE ("Delete")) -> ()
                n381 = local write "Save"(FALSE ("Save")) -> ()
              }
              frame "Query" {
                n382 = local write "Query"(TRUE ("Query")) -> ()
                n383 = local write "Update"(FALSE ("Update")) -> ()
                n384 = local write "Delete"(FALSE ("Delete")) -> ()
                n385 = local write "Save"(FALSE ("Save")) -> ()
                n386 = property on="Luxshare_P/N:" class="Str"("DisabledEnum"=T4."Enabled" ("禁用")) -> ()  [unwired: 2 in, 2 out]
              }
              frame "Update" {
                n387 = local write "Query"(FALSE ("Query")) -> ()
                n388 = local write "Update"(TRUE ("Update")) -> ()
                n389 = local write "Delete"(FALSE ("Delete")) -> ()
                n390 = local write "Save"(FALSE ("Save")) -> ()
                n391 = property on="Luxshare_P/N:" class="Str"("DisabledEnum"=T4."Disabled and Grayed Out" ("禁用")) -> ()  [unwired: 2 in, 2 out]
              }
              frame "Delete" {
                n392 = local write "Query"(FALSE ("Query")) -> ()
                n393 = local write "Update"(FALSE ("Update")) -> ()
                n394 = local write "Delete"(TRUE ("Delete")) -> ()
                n395 = local write "Save"(FALSE ("Save")) -> ()
                n396 = property on="Luxshare_P/N:" class="Str"("DisabledEnum"=T4."Disabled and Grayed Out" ("禁用")) -> ()  [unwired: 2 in, 2 out]
              }
              frame "Save" {
                n397 = local write "Query"(FALSE ("Query")) -> ()
                n398 = local write "Update"(FALSE ("Update")) -> ()
                n399 = local write "Delete"(FALSE ("Delete")) -> ()
                n400 = local write "Save"(TRUE ("Save")) -> ()
                n401 = property on="Luxshare_P/N:" class="Str"("DisabledEnum"=T4."Enabled" ("禁用")) -> ()  [unwired: 2 in, 2 out]
              }
            }
          }
          event "Excute": Value Change {
            n402 = event-data() -> ()  [unwired: 1 in, 5 out]
            n403 = local read "Update"() -> (w470:bool)
            n404 = local read "Query"() -> (w469:bool)
            n405 = local read "Delete"() -> (w468:bool)
            n406 = local read "Save"() -> (w467:bool)
            n407 = call "_wmg_4booltonum.vi"("input4"=w467, "input3"=w468, "input2"=w470, "input1"=w469) -> ("output"=w466:i16)
            n408 = case shown="1000" w466 {
              frame 0, Default {
              }
              frame 1000 {
                n409 = stacked-sequence {
                  frame #0 {
                    n410 = local read "Local"() -> (w471:bool)
                    n411 = case shown="假" w471 {
                      frame True {
                        n412 = stacked-sequence {
                          frame #0 {
                            # "从本地查询，文件一次读取，数据存放在 localQueryResult 中"
                            n413 = local read "Luxshare_P/N:"() -> (w482:string)
                            n414 = Concatenate Strings("Database\\" ("字符串"), w482, ".hpj") -> (w479:string)
                            n415 = call <vilib>:"Application Directory.vi"() -> ("Application Directory"=w480:path)
                            n416 = Build Path(base path=w480, name or relative path=w479) -> (appended path=w478:path)
                            n417 = Read from Binary File(5:string[] [], 9:T7."big-endian, network order" ("字节顺序(0:big-endian, network order)"), 11:w478) -> (0:w473:errorcluster, 2:→"localQueryResult":string[])  [unwired: 3 in, 2 out]
                            n418 = Unbundle(w473) -> ("status"=w472:bool)  [unwired: 2 out]
                            "fileexist" <- w472
                            n419 = case shown="真" w472 {
                              frame False {
                              }
                              frame True {
                                n420 = One Button Dialog(message="请检查文件是否存在") -> ()  [unwired: 1 in, 1 out]
                              }
                            }
                          }
                          frame #1 {
                            # "解析 localQueryResult"
                            n421 = local read "localQueryResult"() -> (w504:string[])
                            n422 = Index Array(array=w504, index #1=0 ("索引"), index #6=5 ("索引"), index #11=10 ("索引")) -> (element #2=w500:string, element #3=w499:string, element #4=w498:string, element #5=w497:string, element #6=w496:string, element #7=w495:string, element #8=w494:string, element #9=w493:string, element #10=w484:string, element #11=w485:string, element #12=w489:string, element #13=w488:string)  [unwired: 10 in, 1 out]
                            n423 = Decimal String To Number(string=w484) -> (number=w490:i32)  [unwired: 2 in, 1 out]
                            n424 = local write "FixtureNo"(w488) -> ()
                            n425 = local write "SNType"(w489) -> ()
                            n426 = Number To Boolean Array(number=w490) -> (Boolean array=w492:bool[])
                            n427 = property on="CmdType" class="Ring (严格)"() -> ("StringsAndValues[]"=w486:T9)  [unwired: 2 in, 2 out]
                            n428 = Index Array(array=w492) -> (element=w491:bool)  [unwired: 1 in]
                            n429 = local write "Customer_P/N:"(w500) -> ()
                            n430 = local write "Customer"(w499) -> ()
                            n431 = local write "Project Information"(w498) -> ()
                            n432 = local write "Sample Description:"(w497) -> ()
                            n433 = local write "AWG"(w496) -> ()
                            n434 = local write "Length(mm):"(w495) -> ()
                            n435 = local write "Spec_midVar"(w494) -> ()
                            n436 = local write "Switch Matrix"(w493) -> ()
                            n437 = local write "EEPROM Write/Read ?"(w491) -> ()
                            n438 = call "_wmg_downlistValue.vi"(1:"Customer"=w485, 2:"Customer"=w486) -> ("Customer"=w487:u16)
                            n439 = local write "CmdType"(w487) -> ()
                          }
                          frame #2 {
                            n440 = local read "localQueryResult"() -> (w527:string[])
                            n441 = Index Array(array=w527, index #1=13 ("索引"), index #4=16 ("索引")) -> (element #1=w521:string, element #2=w520:string, element #3=w519:string, element #4=w518:string, element #5=w514:string, element #6=w509:string, element #7=w508:string, element #8=w507:string, element #9=w506:string)  [unwired: 7 in]
                            n442 = Decimal String To Number(string=w506) -> (number=w505:i32)  [unwired: 2 in, 1 out]
                            n443 = local write "Spec File Path"(w507) -> ()
                            n444 = local write "Switch File Path"(w508) -> ()
                            n445 = Decimal String To Number(string=w521) -> (number=w522:i32)  [unwired: 2 in, 1 out]
                            n446 = local write "Label Num"(w520) -> ()
                            n447 = local write "Label Content"(w519) -> ()
                            n448 = local write "Remark:"(w518) -> ()
                            n449 = Decimal String To Number(string=w514) -> (number=w517:i32)  [unwired: 2 in, 1 out]
                            n450 = Number To Boolean Array(number=w522) -> (Boolean array=w524:bool[])
                            n451 = Number To Boolean Array(number=w517) -> (Boolean array=w516:bool[])
                            n452 = Index Array(array=w524) -> (element=w523:bool)  [unwired: 1 in]
                            n453 = Spreadsheet String To Array(delimiter (Tab)="," ("分隔符(Tab)"), format string="" ("格式字符串"), spreadsheet string=w509, array type (2D Dbl)=string[] []) -> (array=w512:string[])
                            n454 = Index Array(array=w516) -> (element=w515:bool)  [unwired: 1 in]
                            n455 = local write "fre-save"(w512) -> ()
                            n456 = local write "Label Print?"(w523) -> ()
                            n457 = local write "AutoSN"(w515) -> ()
                            n458 = local write "Spec Points"(w505) -> ()
                          }
                          frame #3 {
                            n459 = property on="Cable AWG:" class="Ring (严格)"() -> ("StringsAndValues[]"=w541:T9)  [unwired: 2 in, 2 out]
                            n460 = property on="Customer" class="Ring (严格)"() -> ("StringsAndValues[]"=w543:T9)  [unwired: 2 in, 2 out]
                            n461 = local read "Spec_midVar"() -> (w528:string)
                            n462 = local read "Customer"() -> (w542:string)
                            n463 = local read "AWG"() -> (w540:string)
                            n464 = Search and Replace String(replace all?=TRUE ("替换全部？(F)"), input string=w528, search string="#" ("搜索字符串"), replace string="\t") -> (result string=w536:string)  [unwired: 4 in, 3 out]
                            n465 = call "_wmg_downlistValue.vi"(1:"Customer"=w540, 2:"Customer"=w541) -> ("Customer"=w544:u16)
                            n466 = call "_wmg_downlistValue.vi"(1:"Customer"=w542, 2:"Customer"=w543) -> ("Customer"=w545:u16)
                            n467 = local write "Cable AWG:"(w544) -> ()
                            n468 = local write "Customer"(w545) -> ()
                            n469 = Spreadsheet String To Array(format string="%s" ("格式字符串"), spreadsheet string=w536, array type (2D Dbl)=string[][] []) -> (array=w533:string[][])  [unwired: 1 in]
                            n470 = Fract/Exp String To Number(string=w533) -> (number=w530:dbl[][])  [unwired: 3 in, 1 out]
                            n471 = local write "Spec _Data"(w530) -> ()
                            n472 = Array To Spreadsheet String(delimiter (Tab)="#" ("分隔符(Tab)"), array=w530, 3:"%s" ("格式字符串")) -> (spreadsheet string=w529:string)
                            n473 = local write "Spec String"(w529) -> ()
                          }
                        }
                      }
                      frame False {
                        n474 = stacked-sequence {
                          seq-local: [w563 _ _ _] -> [_ w589 _ _]
                          frame #0 {
                            # "1 2 3 4 5 6 \n10 11"
                            n475 = local read "Luxshare_P/N:"() -> (w576:string)
                            n476 = property on="System_Mode" class="Ring (严格)"() -> ("RingText.Text"=w549:string)  [unwired: 2 in, 2 out]
                            n477 = Array To Spreadsheet String(delimiter (Tab)="," ("分隔符(Tab)"), array=string[] ["LuxsharePN", "CustomerPN", "Customer", "SampleDes", "AWG", "Length", "EEPROMTF", "FixtureNo", "LabelTF", "LabelNum", "Remark", "AutoSN", "FrePoints", "Switch_File_Path", "Spec_File_Path", "Spec_Points", "HardWare_Mode"], 3:"" ("格式字符串")) -> (spreadsheet string=w558:string)
                            n478 = call "_wmg_PNtoPNwhereConnect.vi"("Input"=w576) -> ("Output"=w547:string)
                            n479 = call "_wmg_HardModetoHardModewhereConnect.vi"("Input"=w549) -> ("Output"=w548:string)
                            n480 = Concatenate Strings(w547, w548) -> (w546:string)
                            n481 = call "sql-readinfo_vproject.vi"("操作模式"=T6."查询数据", "查询项目"=w558, "限定条件"=w546) -> ("ConvertToArray"=w575:string[][], "ResultString"=→"result_query":string)  [unwired: 14 in, 9 out]
                            n482 = Index Array(array=w575, index (row)=0 ("索引 (行)")) -> (element=w563:string[])  [unwired: 1 in]
                            n483 = Index Array(array=w563, index #1=1 ("索引"), index #6=6 ("索引")) -> (element #1=w572:string, element #2=→"Customer":string, element #3=w568:string, element #4=→"AWG":string, element #5=w567:string, element #6=w564:string, element #7=w556:string, element #8=w552:string, element #9=w551:string, element #10=w550:string)  [unwired: 8 in]
                            n484 = Decimal String To Number(string=w564) -> (number=w562:i32)  [unwired: 2 in, 1 out]
                            n485 = Decimal String To Number(string=w552) -> (number=w553:i32)  [unwired: 2 in, 1 out]
                            n486 = local write "FixtureNo"(w556) -> ()
                            n487 = local write "Label Num"(w551) -> ()
                            n488 = local write "Remark:"(w550) -> ()
                            n489 = Number To Boolean Array(number=w562) -> (Boolean array=w571:bool[])
                            n490 = Number To Boolean Array(number=w553) -> (Boolean array=w555:bool[])
                            n491 = Index Array(array=w571) -> (element=w570:bool)  [unwired: 1 in]
                            n492 = Index Array(array=w555) -> (element=w554:bool)  [unwired: 1 in]
                            n493 = local write "Customer_P/N:"(w572) -> ()
                            n494 = local write "Sample Description:"(w568) -> ()
                            n495 = local write "Length(mm):"(w567) -> ()
                            n496 = local write "EEPROM Write/Read ?"(w570) -> ()
                            n497 = local write "Label Print?"(w554) -> ()
                          }
                          frame #1 {
                            # "数据库中的cmdType不再使用，\n数据库中的SNType不再使用，代之以标签数据库中的snFormat"
                            n498 = Index Array(array=w589, index #1=11 ("索引"), index #2=12 ("索引")) -> (element #1=w585:string, element #2=w581:string)
                            n499 = Decimal String To Number(string=w585) -> (number=w586:i32)  [unwired: 2 in, 1 out]
                            n500 = Number To Boolean Array(number=w586) -> (Boolean array=w587:bool[])
                            n501 = Spreadsheet String To Array(delimiter (Tab)="," ("分隔符(Tab)"), format string="" ("格式字符串"), spreadsheet string=w581, array type (2D Dbl)=string[] []) -> (array=w580:string[])
                            n502 = Index Array(array=w587) -> (element=w584:bool)  [unwired: 1 in]
                            n503 = local write "fre-save"(w580) -> ()
                            n504 = local write "AutoSN"(w584) -> ()
                          }
                          frame #2 {
                            n505 = local read "Luxshare_P/N:"() -> (w627:string)
                            n506 = local read "Luxshare_P/N:"() -> (w630:string)
                            n507 = local read "Luxshare_P/N:"() -> (w633:string)
                            n508 = call "_wmg_PNtoPNwhereConnect.vi"("Input"=w627) -> ("Output"=w601:string)
                            n509 = call "_wmg_PNtoPNwhereConnect.vi"("Input"=w633) -> ("Output"=w606:string)
                            n510 = call "_wmg_PNtoPNwhereConnect.vi"("Input"=w630) -> ("Output"=w604:string)
                            n511 = property on="System_Mode" class="Ring (严格)"() -> ("RingText.Text"=w600:string)  [unwired: 2 in, 2 out]
                            n512 = call "_wmg_HardModetoHardModewhereConnect.vi"("Input"=w600) -> ("Output"=w591:string)
                            n513 = Concatenate Strings(w606, w591) -> (w605:string)
                            n514 = call "sql-readinfo_vproject.vi"("操作模式"=T6."查询数据", "查询项目"="Prjinf", "限定条件"=w605) -> ("ResultString"=w620:string)  [unwired: 14 in, 10 out]
                            n515 = local write "Project Information"(w620) -> ()
                            n516 = Concatenate Strings(w601, w591) -> (w599:string)
                            n517 = call "sql-readinfo_vproject.vi"("操作模式"=T6."查询数据", "查询项目"="SwitchMatrix", "限定条件"=w599) -> ("ResultString"=w622:string)  [unwired: 14 in, 10 out]
                            n518 = Concatenate Strings(w604, w591) -> (w603:string)
                            n519 = call "sql-readinfo_vproject.vi"("操作模式"=T6."查询数据", "查询项目"="Spec", "限定条件"=w603) -> ("ResultString"=→"Spec_midVar":string)  [unwired: 14 in, 10 out]
                            n520 = local write "Switch Matrix"(w622) -> ()
                            n521 = local read "Luxshare_P/N:"() -> (w612:string)
                            n522 = local read "Luxshare_P/N:"() -> (w615:string)
                            n523 = local read "Luxshare_P/N:"() -> (w618:string)
                            n524 = local read "Luxshare_P/N:"() -> (w624:string)
                            n525 = call "_wmg_PNtoPNwhereConnect.vi"("Input"=w612) -> ("Output"=w592:string)
                            n526 = Concatenate Strings(w592, w591) -> (w590:string)
                            n527 = call "_wmg_PNtoPNwhereConnect.vi"("Input"=w615) -> ("Output"=w594:string)
                            n528 = Concatenate Strings(w594, w591) -> (w593:string)
                            n529 = call "_wmg_PNtoPNwhereConnect.vi"("Input"=w618) -> ("Output"=w596:string)
                            n530 = Concatenate Strings(w596, w591) -> (w595:string)
                            n531 = call "sql-readinfo_vproject.vi"("操作模式"=T6."查询数据", "查询项目"="Spec_Points", "限定条件"=w590) -> ("ResultString"=w608:string)  [unwired: 14 in, 10 out]
                            n532 = call "sql-readinfo_vproject.vi"("操作模式"=T6."查询数据", "查询项目"="Switch_File_Path", "限定条件"=w595) -> ("ResultString"=w610:string)  [unwired: 14 in, 10 out]
                            n533 = call "_wmg_PNtoPNwhereConnect.vi"("Input"=w624) -> ("Output"=w598:string)
                            n534 = Concatenate Strings(w598, w591) -> (w597:string)
                            n535 = call "sql-readinfo_vproject.vi"("操作模式"=T6."查询数据", "查询项目"="LabelC", "限定条件"=w597) -> ("ResultString"=w621:string)  [unwired: 14 in, 10 out]
                            n536 = call "sql-readinfo_vproject.vi"("操作模式"=T6."查询数据", "查询项目"="Spec_File_Path", "限定条件"=w593) -> ("ResultString"=w609:string)  [unwired: 14 in, 10 out]
                            n537 = local write "Switch File Path"(w610) -> ()
                            n538 = Decimal String To Number(string=w608) -> (number=w607:i32)  [unwired: 2 in, 1 out]
                            n539 = local write "Spec Points"(w607) -> ()
                            n540 = local write "Spec File Path"(w609) -> ()
                            n541 = local write "Label Content"(w621) -> ()
